vi "Read Measured Value.vi"(7 "unit (capacity unit)":u16(ring) items=["capacity unit", "%"], 8 "error in (no error)":errorcluster, 10 "node address (same)":u8, 11 "ProPar in":refnum<class "PL Bronkhorst ProPar.lvclass">) -> (0 "error out":errorcluster, 2 "measured value":sgl, 3 "ProPar out":refnum<class "PL Bronkhorst ProPar.lvclass">)   [LabVIEW 2015, in "PL Bronkhorst ProPar.lvclass"]
doc: "Reads measured value of the specified <b>node</b>."
uses:
  PL Bronkhorst ProPar.lvclass
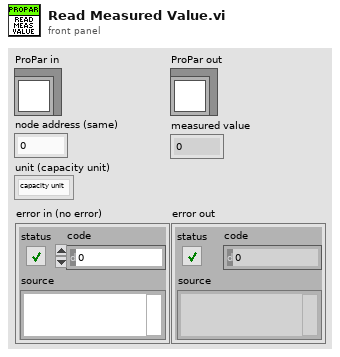
[diagram p1: front panel]
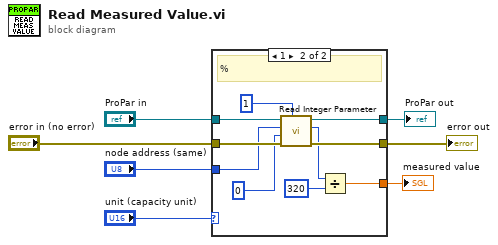
[diagram p0: block diagram]
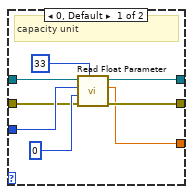
[diagram p2: hidden frame]
diagram:
  n1 = case shown="1" "unit (capacity unit)" {
    tunnel: [w14 w21] -> w7
    tunnel: [w13 w20] -> w6
    tunnel: "ProPar in" -> [w12 w23]
    tunnel: "node address (same)" -> [w11 w18]
    tunnel: [w9 w25] -> w3
    tunnel: "error in (no error)" -> [w8 w22]
    frame 0, Default {
      # "capacity unit"
      n2 = call "Read Float Parameter.vi"("process number"=u8 33, "error in (no error)"=w8, "parameter number"=u8 0 ("process number"), "node"=w11, "ProPar in"=w12) -> ("error out"=w14:errorcluster, "value"=w9:sgl, "ProPar out"=w13:refnum<class "PL Bronkhorst ProPar.lvclass">)  [unwired: 4 in]
    }
    frame 1 {
      # "%"
      n3 = call "Read Integer Parameter.vi"("process number"=u8 1, "error in (no error)"=w22, "parameter number"=u8 0 ("process number"), "node"=w18, "ProPar in"=w23) -> ("error out"=w21:errorcluster, "value"=w19:u16, "ProPar out"=w20:refnum<class "PL Bronkhorst ProPar.lvclass">)  [unwired: 4 in]
      n4 = Divide(x=w19, y=u16 320) -> (x/y=w25:dbl)
    }
  }
  "ProPar out" <- w6
  "error out" <- w7
  "measured value" <- w3
